vi "GetMeasurementsGroups.vi"(8 "error in (no error)":errorcluster, 10 "id (-1 ReadAll)":i32=-1, 11 "ByteGSAPIBase in":refnum<class "ByteGSAPIBase.lvclass">) -> (0 "error out":errorcluster, 2 "measurements":T1, 3 "ByteGSAPIBase out":refnum<class "ByteGSAPIBase.lvclass">)   [LabVIEW 2019, in "ByteGSWebAPI.lvlib" / "ByteGSAPIBase.lvclass"]
doc: "Obtain data for measurements based on the id"
uses:
  ByteGSAPIBase.lvclass
  ByteGSAPIBase.lvclass/ByteGSAPIBase.ctl
  <vilib>/Bytelabs/ByteREST/ByteRESTClass/ByteRESTBase/RESTBase.lvclass
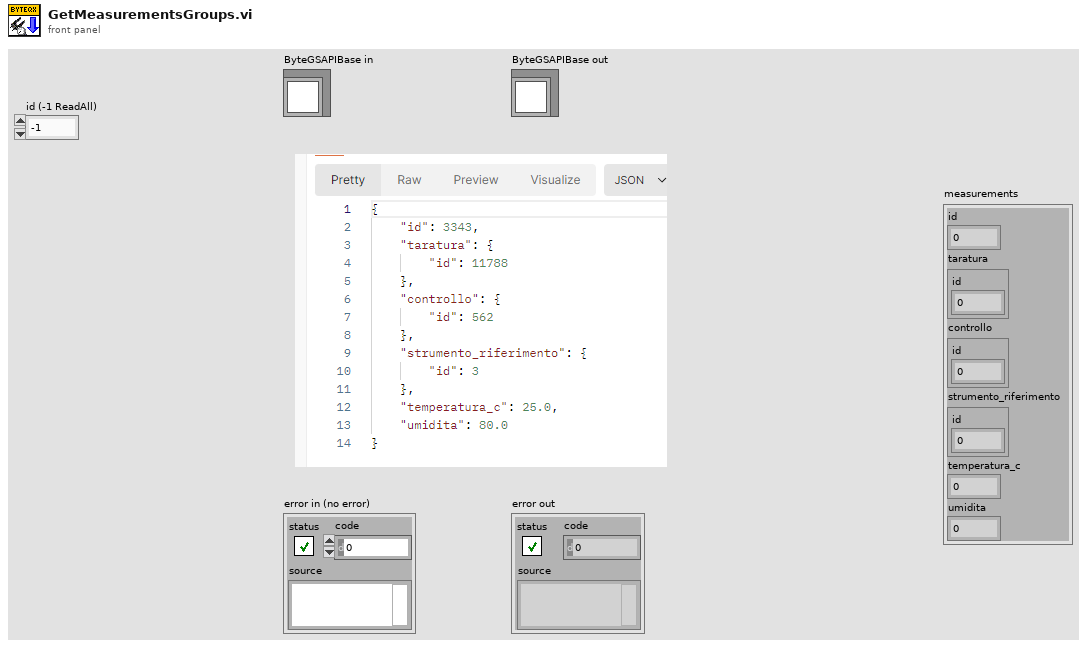
[diagram p1: front panel]
types:
  T1 = cluster{"id":u32, "taratura":cluster{"id":u32}, "controllo":cluster{"id":u32}, "strumento_riferimento":cluster{"id":u32}, "temperatura_c":u32, "umidita":u32}
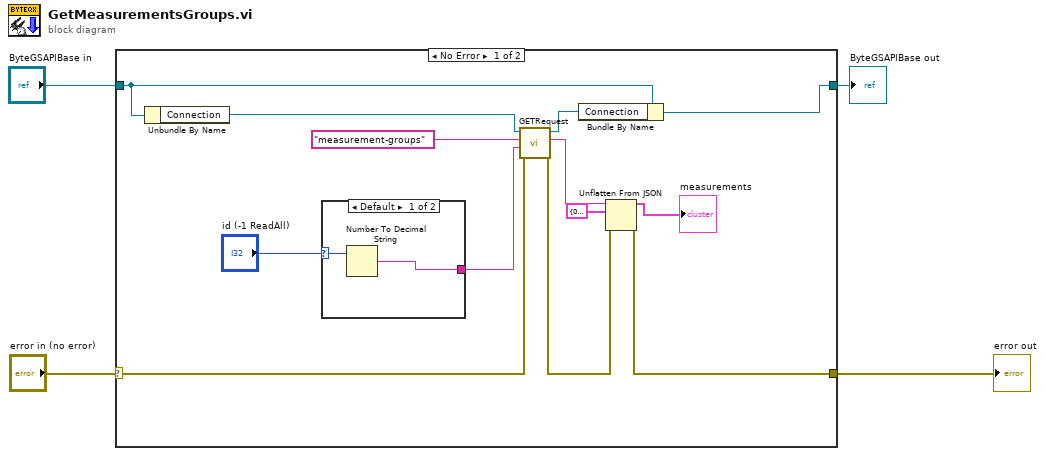
[diagram p0: block diagram]
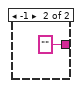
[diagram p2: hidden frame]
diagram:
  n1 = case shown="No Error" "error in (no error)" {
    selector: "error in (no error)" -> [w10 w22]
    tunnel: [w9 w22] -> w2
    tunnel: [w14 w21] -> w3
    tunnel: "ByteGSAPIBase in" -> [w17 w21]
    frame No Error {
      n2 = Unbundle By Name(w17) -> ("Connection"=w16:refnum<class "RESTBase.lvclass">)
      n3 = case shown="Default" "id (-1 ReadAll)" {
        selector: "id (-1 ReadAll)" -> [w19 _]
        tunnel: [w18 ""] -> w7
        frame Default {
          n4 = Number To Decimal String(number=w19) -> (decimal integer string=w18:string)  [unwired: 1 in]
        }
        frame -1 {
        }
      }
      n5 = call-dynamic "GETRequest.vi"("error in (no error)"=w10, "Parameter"=w7, "Request"="measurement-groups", "ByteRESTBase in"=w16) -> ("error out"=w15:errorcluster, "Body"=w11:string, "ByteRESTBase out"=w13:refnum<class "RESTBase.lvclass">)  [unwired: 4 in, 1 out]
      n6 = Bundle By Name(cluster=w17, "Connection"=w13) -> (w14:refnum<class "ByteGSAPIBase.lvclass">)
      n7 = Unflatten From JSON(JSON string=w11, type and defaults=T1 {"id"=0, "taratura"={"id"=0}, "controllo"={"id"=0}, "strumento_riferimento"={"id"=0}, "temperatura_c"=0, "umidita"=0} ("Cluster 2"), error in (no error)=w15) -> (value=→"measurements":T1, error out=w9:errorcluster)  [unwired: 4 in]
    }
    frame Error {
    }
  }
  "error out" <- w2
  "ByteGSAPIBase out" <- w3
